vi "Start Running.vi"(8 "error in (no error)":errorcluster, 11 "CIFCorePlugin in":refnum<class "CIFCorePlugin.lvclass">) -> (0 "error out":errorcluster, 3 "CIFCorePlugin out":refnum<class "CIFCorePlugin.lvclass">)   [LabVIEW 2021, in "CIFCorePlugin.lvclass"]
doc: "Update the timestamp. Time is U64, absolute time in nS in the appropriate clockID configured for the plugin. If a 0 is wired it will automatically get the current time."
uses:
  CIFCorePlugin.lvclass
  CIFCorePlugin.lvclass/CIFCorePlugin.ctl
  CIFUtilities/CIFClocks/Typedef/Future Time Event Limits.ctl
  CIFUtilities/CIFClocks/Time Conversion/LabVIEW Time to UTC Time.vi
  CIFUtilities/CIFClocks/SubVIs/Add Error.vi
  CIFUtilities/CIFClocks/CIFClocks.lvlib
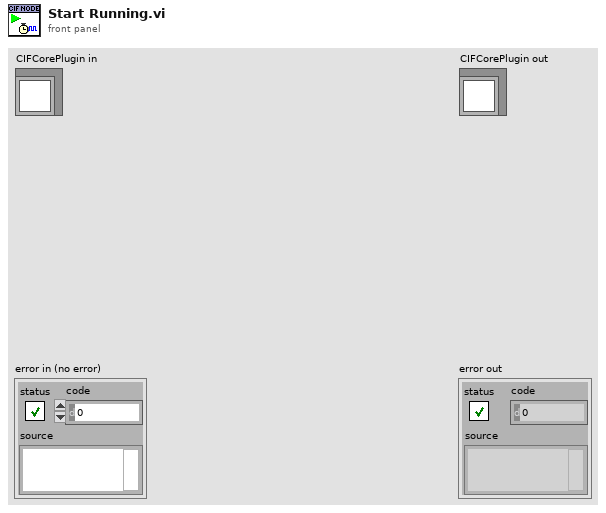
[diagram p1: front panel]
types:
  T1 = typedef "CIFClocks.lvlib/Future Time Event Limits.ctl" = cluster{"Maximum":u64, "Minimum":u64}
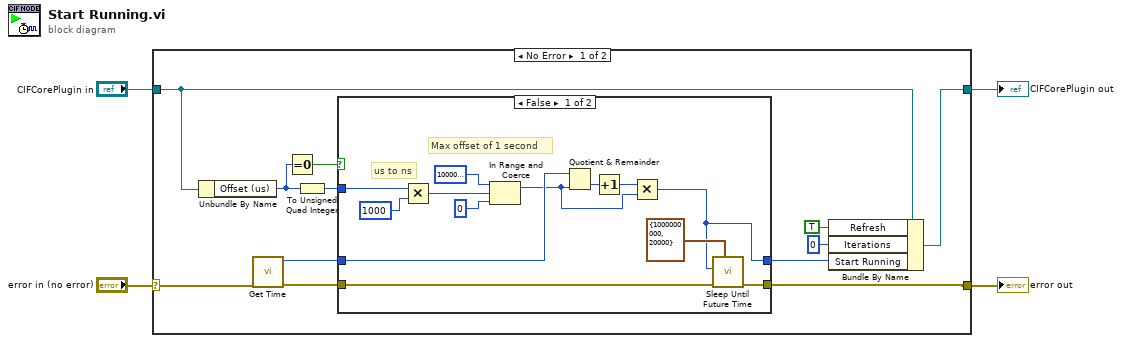
[diagram p0: block diagram]
diagram:
  n1 = case shown="No Error" "error in (no error)" {
    selector: "error in (no error)" -> [w14 w32]
    tunnel: [w7 w32] -> w3
    tunnel: [w16 w33] -> w1
    tunnel: "CIFCorePlugin in" -> [w15 w33]
    frame No Error {
      n2 = Unbundle By Name(w15) -> ("Offset (us)"=w10:i32)
      n3 = call "Get Time.vi"("error in (no error)"=w14) -> ("error out"=w8:errorcluster, "Time (ns)"=w13:u64)  [unwired: 8 in, 1 out]
      n4 = Equal To 0?(x=w10) -> (x = 0?=w11:bool)
      n5 = To Unsigned Quad Integer(1:w10) -> (0:w9:u64)
      n6 = case shown="False" w11 {
        tunnel: w13 -> [w27 w31]
        tunnel: [w17 w31] -> w12
        tunnel: w9 -> [w23 _]
        tunnel: w8 -> [w25 w30]
        tunnel: [w24 w30] -> w7
        frame False {
          # "us to ns"
          # "Max offset of 1 second"
          n7 = Multiply(x=w23, y=u64 1000) -> (x*y=w21:u64)
          n8 = In Range and Coerce(upper limit=u64 1000000000, x=w21, lower limit=u64 0) -> (coerced(x)=w18:u64)  [unwired: 1 out]
          n9 = Quotient & Remainder(x=w27, y=w18) -> (floor(x/y)=w20:u64)  [unwired: 1 out]
          n10 = Increment(x=w20) -> (x+1=w19:u64)
          n11 = Multiply(x=w19, y=w18) -> (x*y=w17:u64)
          n12 = call "Sleep Until Future Time.vi"("FTE Limits (ns)"=T1 {"Maximum"=1000000000, "Minimum"=20000}, "error in (no error)"=w25, "Wake Time"=w17) -> ("error out"=w24:errorcluster)  [unwired: 8 in]
        }
        frame True {
        }
      }
      n13 = Bundle By Name(cluster=w15, "Refresh"=TRUE, "Iterations"=i64 0, "Start Running"=w12) -> (w16:refnum<class "CIFCorePlugin.lvclass">)
    }
    frame Error {
    }
  }
  "error out" <- w3
  "CIFCorePlugin out" <- w1
